vi "LNG Boiling Front Panel.vi"() -> ()   [LabVIEW 2019, in "Results.lvlib" / "LNG Boiling Results.lvclass"]
uses:
  LNG Boiling Results.lvclass
  LNG Boiling Results.lvclass/LNG Boiling Results.ctl
  Test Stands/LNG Boiling/LNG Boiling Test Stand.lvclass
panel:
  out "Adjusted":bool
  in  "Htr Temp SP":dbl=292.0 caption="Heater Temperature" min=0.0 max=372.0 step=1.0
  in  "auto Temp":bool
  in  "Htr MOS Ctrl":dbl caption="Heater MOS Control" min=0.0 max=10.0 step=0.1
  in  "Htr Pwr SP":dbl caption="Heater Power" min=0.0 max=300.0 step=1.0
  out "Heater Power":dbl(slide) scale=0.0..100.0
  in  "auto pwr":bool
  out "Heater dU":dbl format="%#.3f"
  out "Shunt dU":dbl format="%#.4f"
  out "aslant":dbl format="%#.2f"
  out "outer":dbl format="%#.2f"
  out "inner":dbl format="%#.2f"
  out "above":dbl format="%#.2f"
  out "inside":dbl format="%#.2f"
  out "I":dbl format="%#.3f"
  out "P":dbl format="%#.3f"
  out "Data":waveform(dbl)[](graph) caption="Temperatures"
  # "Automatic"
  # "A"
  # "W"
  # "Manual"
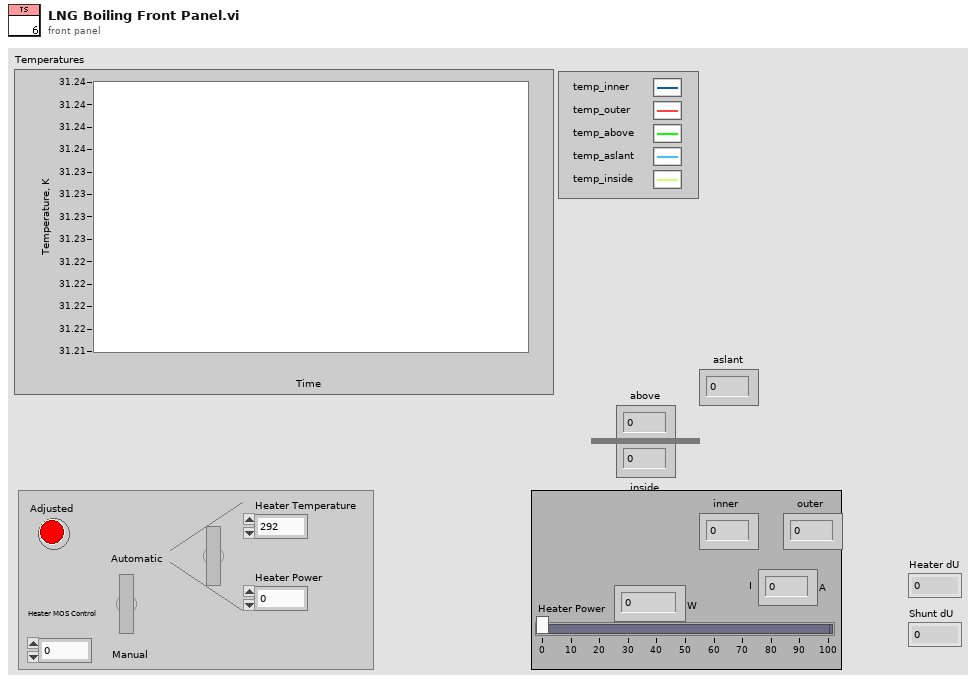
[diagram p1: front panel]
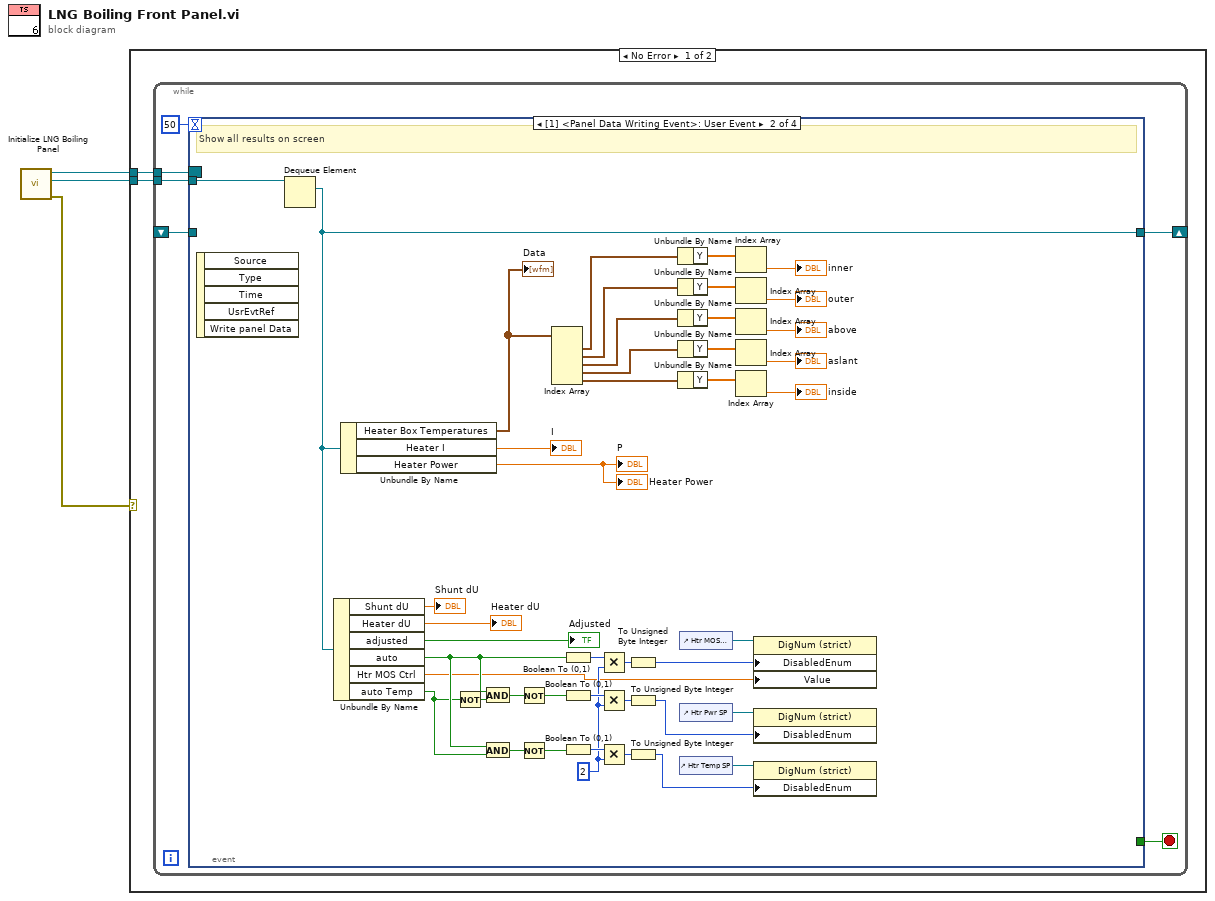
[diagram p0: block diagram]
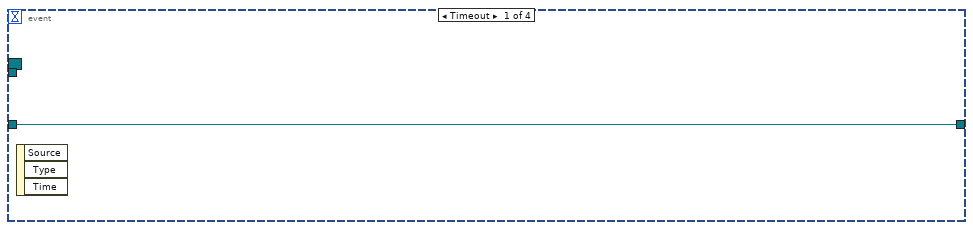
[diagram p2: hidden frame]
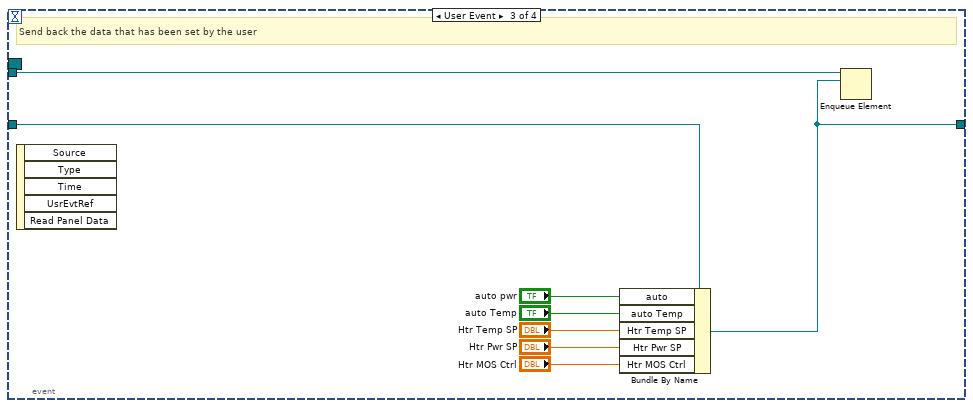
[diagram p3: hidden frame]
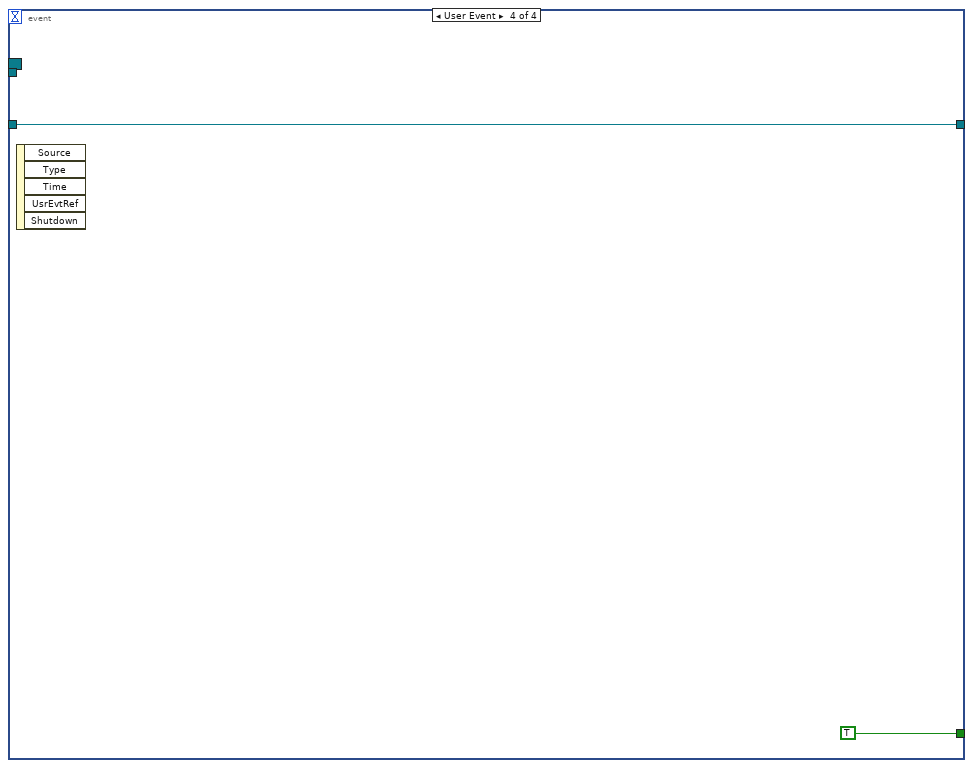
[diagram p4: hidden frame]
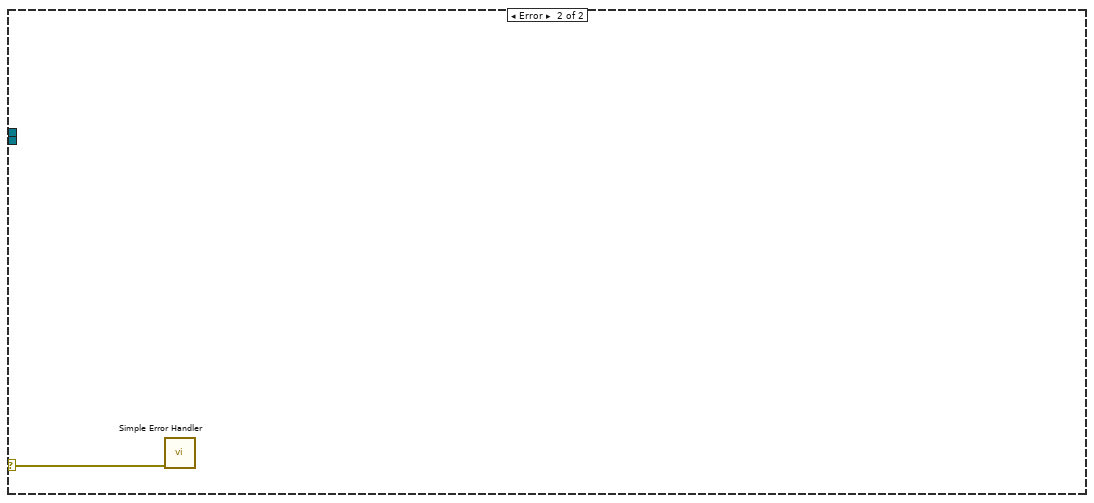
[diagram p5: hidden frame]
diagram:
  n1 = call "Initialize LNG Boiling Panel.vi"() -> ("error out"=w3:errorcluster, "LNG Boiling Results queue out"=w1:refnum<queue>, "Event Registration Refnum"=w2:refnum<event-registration>)  [unwired: 9 in]
  n2 = case shown="No Error" w3 {
    selector: w3 -> [_ w67]
    tunnel: w2 -> [w5 _]
    tunnel: w1 -> [w4 _]
    frame No Error {
      n3 = while {
        tunnel: w5 -> [w10]
        tunnel: w4 -> [w9]
        shift-right: [w7] -> _
        shift-left: _ -> [w6]
        stop <- w11 stop-if-true
        n4 = event shown="[1] <Panel Data Writing Event>: User Event" {
          selector: w10 -> [_ _ _ _]
          dyn-events: _ -> [_ _ _ _]
          timeout: 50 -> [_ _ _ _]
          tunnel: [_ _ _ TRUE] -> w11
          tunnel: w9 -> [_ w56 w64 _]
          tunnel: [w12 w38 w62 w65] -> w7
          tunnel: w6 -> [w12 _ w63 w65]
          event Timeout {
            n5 = event-data() -> ()  [unwired: 1 in, 3 out]
          }
          event User Event {
            w15 = i16 2 ("y")
            # "Show all results on screen"
            n6 = event-data() -> ()  [unwired: 1 in, 5 out]
            n7 = Dequeue Element(queue=w56) -> (element=w38:refnum<class "LNG Boiling Results.lvclass">)  [unwired: 2 in, 3 out]
            n8 = Unbundle By Name(w38) -> ("Shunt dU"=→"Shunt dU":dbl, "Heater dU"=→"Heater dU":dbl, "adjusted"=→"Adjusted":bool, "auto"=w19:bool, "Htr MOS Ctrl"=w14:dbl, "auto Temp"=w16:bool)
            n9 = Unbundle By Name(w38) -> ("Heater Box Temperatures"=w55:waveform(dbl)[], "Heater I"=→"I":dbl, "Heater Power"=→"P" →"Heater Power":dbl)
            "Data" <- w55
            n10 = Not(x=w16) -> (.not. x?=w29:bool)
            n11 = And(x=w19, y=w29) -> (x .and. y?=w28:bool)
            n12 = And(x=w19, y=w16) -> (x .and. y?=w20:bool)
            n13 = Not(x=w28) -> (.not. x?=w24:bool)
            n14 = Not(x=w20) -> (.not. x?=w18:bool)
            n15 = Index Array(array=w55) -> (element #1=w54:waveform(dbl), element #2=w51:waveform(dbl), element #3=w48:waveform(dbl), element #4=w46:waveform(dbl), element #5=w44:waveform(dbl))  [unwired: 5 in]
            n16 = Boolean To (0,1)(Boolean=w19) -> (0, 1=w32:i16)
            n17 = Boolean To (0,1)(Boolean=w24) -> (0, 1=w26:i16)
            n18 = Boolean To (0,1)(Boolean=w18) -> (0, 1=w23:i16)
            n19 = Multiply(x=w32, y=w15) -> (x*y=w31:i16)
            n20 = Multiply(x=w26, y=w15) -> (x*y=w27:i16)
            n21 = Multiply(x=w23, y=w15) -> (x*y=w22:i16)
            n22 = To Unsigned Byte Integer(number=w31) -> (unsigned 8bit integer=w30:u8)
            n23 = To Unsigned Byte Integer(number=w27) -> (unsigned 8bit integer=w25:u8)
            n24 = To Unsigned Byte Integer(number=w22) -> (unsigned 8bit integer=w21:u8)
            n25 = Unbundle By Name(w54) -> ("Y"=w53:dbl[])
            n26 = Unbundle By Name(w51) -> ("Y"=w50:dbl[])
            n27 = Unbundle By Name(w48) -> ("Y"=w47:dbl[])
            n28 = Unbundle By Name(w46) -> ("Y"=w45:dbl[])
            n29 = Unbundle By Name(w44) -> ("Y"=w43:dbl[])
            n30 = control-ref of="Htr MOS Ctrl"() -> (w33:refnum<vi>)
            n31 = control-ref of="Htr Pwr SP"() -> (w17:refnum<vi>)
            n32 = control-ref of="Htr Temp SP"() -> (w13:refnum<vi>)
            n33 = Index Array(array=w53) -> (element=→"inner":dbl)  [unwired: 1 in]
            n34 = Index Array(array=w50) -> (element=→"outer":dbl)  [unwired: 1 in]
            n35 = Index Array(array=w47) -> (element=→"above":dbl)  [unwired: 1 in]
            n36 = Index Array(array=w45) -> (element=→"aslant":dbl)  [unwired: 1 in]
            n37 = Index Array(array=w43) -> (element=→"inside":dbl)  [unwired: 1 in]
            n38 = property class="DigNum (strict)"(reference=w33, "DisabledEnum"=w30, "Value"=w14) -> ()  [unwired: 1 in, 2 out]
            n39 = property class="DigNum (strict)"(reference=w17, "DisabledEnum"=w25) -> ()  [unwired: 1 in, 2 out]
            n40 = property class="DigNum (strict)"(reference=w13, "DisabledEnum"=w21) -> ()  [unwired: 1 in, 2 out]
          }
          event User Event {
            # "Send back the data that has been set by the user"
            n41 = event-data() -> ()  [unwired: 1 in, 5 out]
            n42 = Bundle By Name(cluster=w63, "auto"="auto pwr", "auto Temp"="auto Temp", "Htr Temp SP"="Htr Temp SP", "Htr Pwr SP"="Htr Pwr SP", "Htr MOS Ctrl"="Htr MOS Ctrl") -> (w62:refnum<class "LNG Boiling Results.lvclass">)
            n43 = Enqueue Element(queue=w64, element=w62) -> ()  [unwired: 2 in, 3 out]
          }
          event User Event {
            n44 = event-data() -> ()  [unwired: 1 in, 5 out]
          }
        }
      }
    }
    frame Error {
      n45 = call <vilib>:"Simple Error Handler.vi"("error in (no error)"=w67) -> ()  [unwired: 4 in, 5 out]
    }
  }
